vi "Handle Last Ack Core.vi"(4 "error in (no error)":errorcluster, 6 "Last Ack":refnum<class "Last Ack.lvclass">, 7 "Function in":refnum<class "Function.lvclass">) -> (0 "error out":errorcluster, 3 "Function out":refnum<class "Function.lvclass">)   [LabVIEW 2016, in "Function Actor.lvlib" / "Function.lvclass"]
doc: "(<B>Filename</B>: Actor Framework.lvlib:Actor.lvclass:Handle Last Ack Core.vi)\n\nDefines how the caller actor responds to the Last Ack message from a nested actor. The Last Ack message is the final message a nested actor sends to its caller before it shuts down. The message contains information about the final state of the nested actor.\n\nBy default, this method does nothing except return any error the nested actor sent. A descendant class may override this method to define behavior."
uses:
  <userlib>/Common Components/Function Actor/Function.lvclass
  <vilib>/ActorFramework/LastAck/Last Ack.lvclass
  <vilib>/ActorFramework/LastAck/Last Ack.lvclass/Last Ack.ctl
  <userlib>/Configuration Dialog Actor/Configuration.lvclass
  <userlib>/Configuration Dialog Actor/Configuration.lvclass/Configuration.ctl
  <userlib>/Common Components/Function Actor/Function.lvclass/Function.ctl
  <vilib>/ActorFramework/Actor/Actor.lvclass
  <userlib>/Common Components/Controller/Controller.lvclass
  C:/Program Files (x86)/National Instruments/LabVIEW 2016/vi.lib/ActorFramework/Actor/Actor.lvclass
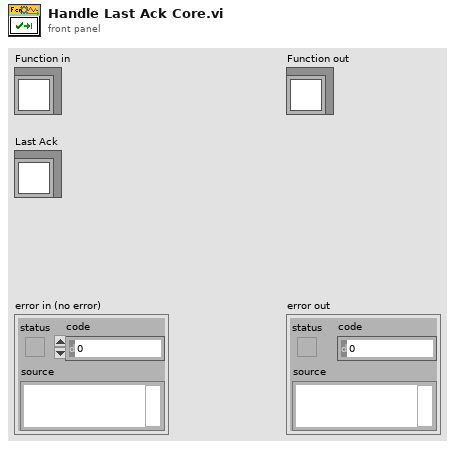
[diagram p1: front panel]
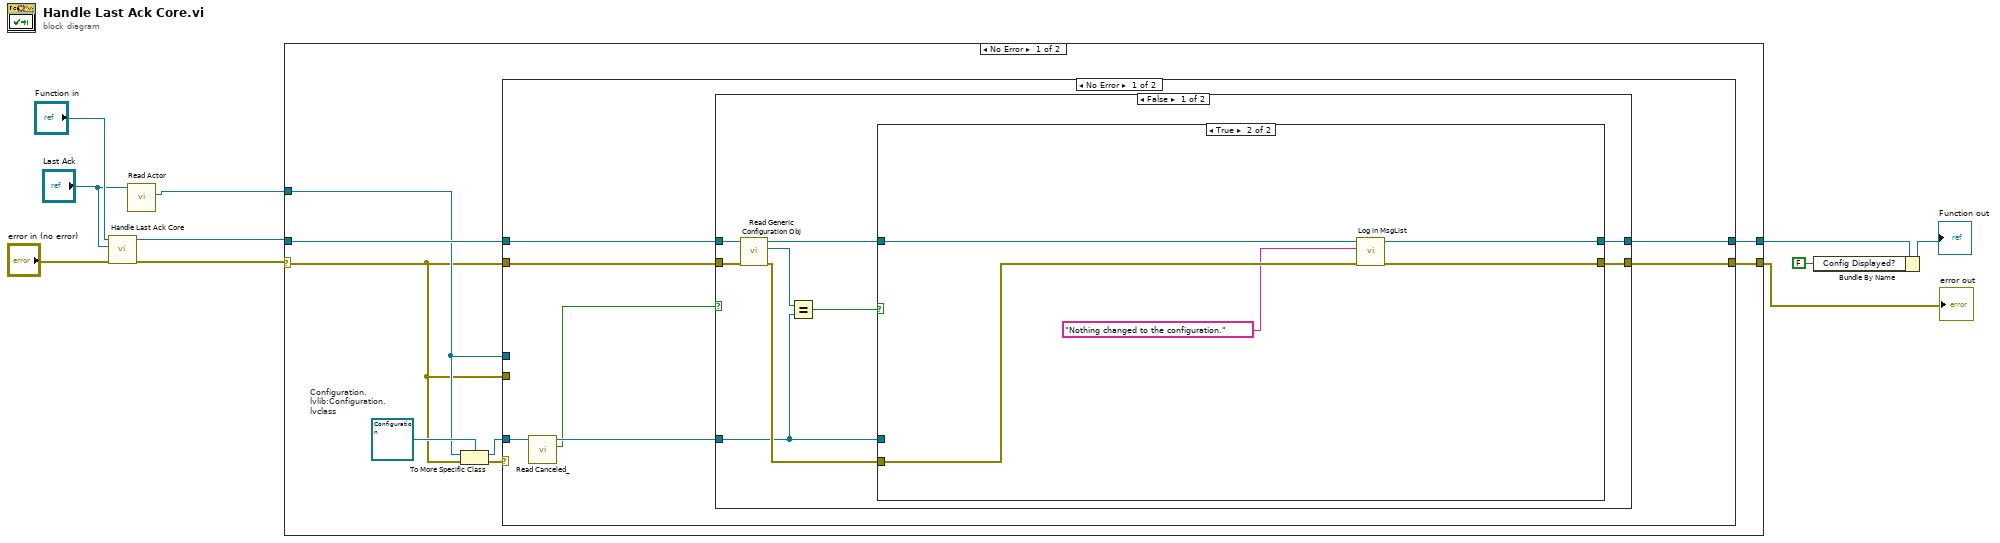
[diagram p0: block diagram]
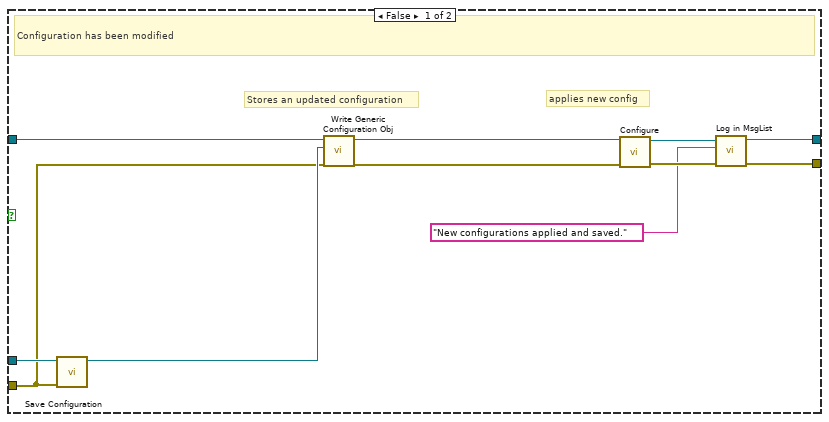
[diagram p2: hidden frame]
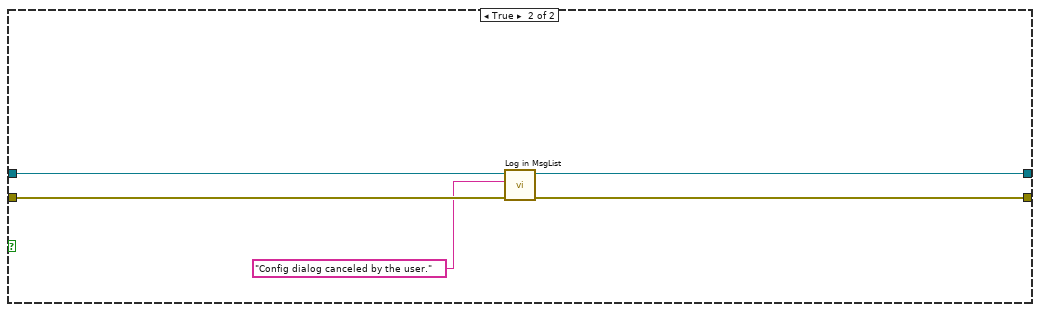
[diagram p3: hidden frame]
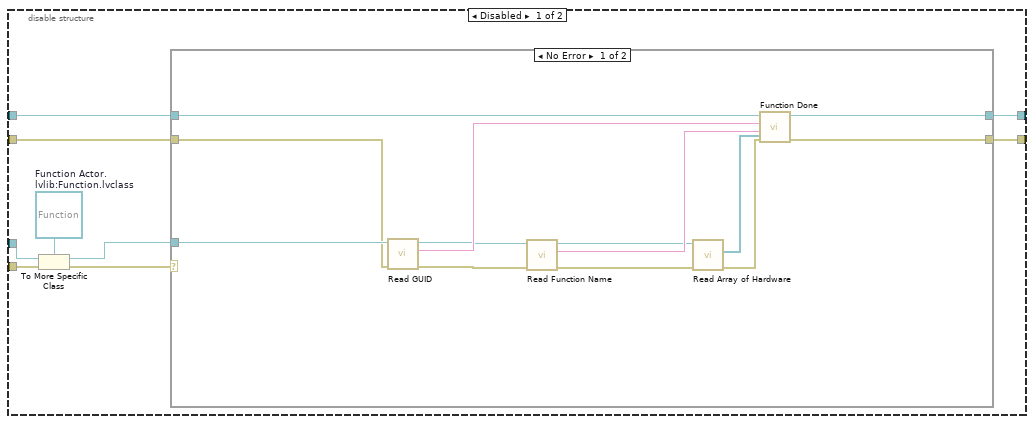
[diagram p5: hidden frame]
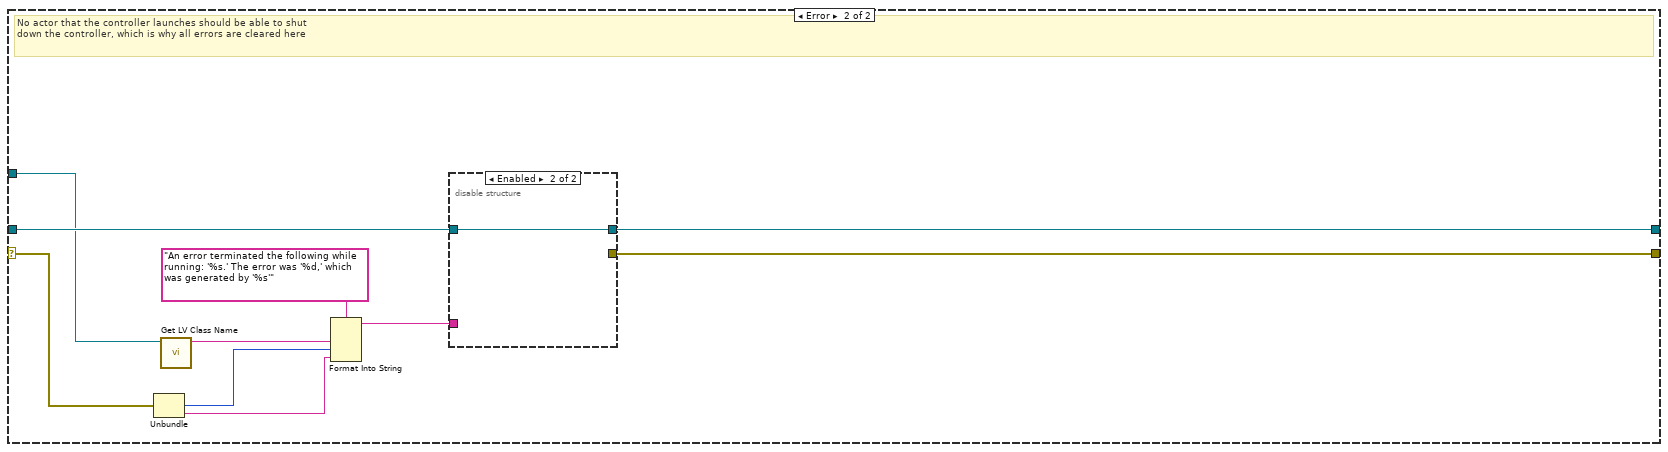
[diagram p7: hidden frame]
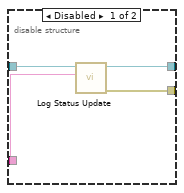
[diagram p8: hidden frame]
diagram:
  n1 = call-parent "Handle Last Ack Core.vi"("error in (no error)"="error in (no error)", "Last Ack"="Last Ack", "Actor in"="Function in") -> ("error out"=w5:errorcluster, "Actor out"=w6:refnum<class "Function.lvclass">)  [unwired: 3 in]
  n2 = call <vilib>:"Read Actor.vi"("Last Ack"="Last Ack") -> ("Actor"=w7:refnum<class "Actor.lvclass">)  [unwired: 10 in]
  n3 = case shown="No Error" w5 {
    selector: w5 -> [w11 w92]
    tunnel: [w18 w95] -> w3
    tunnel: [w17 w94] -> w4
    tunnel: w6 -> [w16 w96]
    tunnel: w7 -> [w12 w88]
    frame No Error {
      w13 = refnum<class "Configuration.lvclass"> refnum  # Configuration.lvlib:Configuration.lvclass
      n4 = To More Specific Class(target class=w13, reference=w12, error in=w11) -> (specific class reference=w15:refnum<class "Configuration.lvclass">, error out=w14:errorcluster)
      n5 = case shown="No Error" w14 {
        tunnel: [w21 w56] -> w18
        tunnel: [w25 w55] -> w17
        tunnel: w16 -> [w24 w58]
        tunnel: w15 -> [w22 _]
        tunnel: w11 -> [w23 w57]
        tunnel: w12 -> [_ w60]
        tunnel: w11 -> [_ w59]
        frame No Error {
          n6 = call <vilib>:"Read Canceled_.vi"("Configuration in"=w22) -> ("Canceled?"=w19:bool, "Configuration out"=w20:refnum<class "Configuration.lvclass">)  [unwired: 8 in, 1 out]
          n7 = case shown="False" w19 {
            tunnel: [w34 w53] -> w25
            tunnel: w24 -> [w33 w52]
            tunnel: w23 -> [w29 w54]
            tunnel: [w27 w51] -> w21
            tunnel: w20 -> [w26 _]
            frame False {
              n8 = call <userlib>:"Read Generic Configuration Obj.vi"("error in (no error)"=w29, "Function in"=w33) -> ("error out"=w32:errorcluster, "Configuration.lvlib:Configuration.lvclass"=w31:refnum<class "Configuration.lvclass">, "Function out"=w28:refnum<class "Function.lvclass">)  [unwired: 7 in]
              n9 = Equal?(x=w31, y=w26) -> (x = y?=w30:bool)
              n10 = case shown="True" w30 {
                tunnel: w26 -> [w44 _]
                tunnel: w32 -> [w40 w49]
                tunnel: w28 -> [w42 w47]
                tunnel: [w36 w46] -> w27
                tunnel: [w38 w48] -> w34
                frame False {
                  # "applies new config"
                  # "Stores an updated configuration"
                  # "Configuration has been modified"
                  n11 = call <userlib>:"Save Configuration.vi"("error in (no error)"=w40, "Configuration in"=w44) -> ("Configuration out"=w43:refnum<class "Configuration.lvclass">)  [unwired: 7 in, 2 out]
                  n12 = call <userlib>:"Write Generic Configuration Obj.vi"("Configuration.lvlib:Configuration.lvclass"=w43, "Function in"=w42) -> ("Function out"=w41:refnum<class "Function.lvclass">)  [unwired: 8 in, 1 out]
                  n13 = call-dynamic "Configure.vi"("error in (no error)"=w40, "Function in"=w41) -> ("error out"=w39:errorcluster, "Function out"=w37:refnum<class "Function.lvclass">)  [unwired: 8 in]
                  n14 = call-dynamic "Log in MsgList.vi"("error in (no error)"=w39, "Msg"="New configurations applied and saved.", "Function in"=w37) -> ("error out"=w38:errorcluster, "Function out"=w36:refnum<class "Function.lvclass">)  [unwired: 7 in]
                }
                frame True {
                  n15 = call-dynamic "Log in MsgList.vi"("error in (no error)"=w49, "Msg"="Nothing changed to the configuration.", "Function in"=w47) -> ("error out"=w48:errorcluster, "Function out"=w46:refnum<class "Function.lvclass">)  [unwired: 7 in]
                }
              }
            }
            frame True {
              n16 = call-dynamic "Log in MsgList.vi"("error in (no error)"=w54, "Msg"="Config dialog canceled by the user.", "Function in"=w52) -> ("error out"=w53:errorcluster, "Function out"=w51:refnum<class "Function.lvclass">)  [unwired: 7 in]
            }
          }
        }
        frame Error {
          n17 = disable-structure shown="Enabled" {
            disable-tunnel: w60 -> [w69 _]
            disable-tunnel: w59 -> [w68 _]
            disable-tunnel: w58 -> [w64 w86]
            disable-tunnel: w57 -> [w63 w85]
            disable-tunnel: [w62 w86] -> w56
            disable-tunnel: [w61 w85] -> w55
            frame Disabled {
              w67 = refnum<class "Function.lvclass"> refnum  # Function Actor.lvlib:Function.lvclass
              n18 = To More Specific Class(target class=w67, reference=w69, error in=w68) -> (specific class reference=w65:refnum<class "Function.lvclass">, error out=w66:errorcluster)
              n19 = case shown="No Error" w66 {
                tunnel: w65 -> [w76 _]
                tunnel: w64 -> [w82 w84]
                tunnel: w63 -> [w72 w83]
                tunnel: [w81 w84] -> w62
                tunnel: [w80 w83] -> w61
                frame No Error {
                  n20 = call <userlib>:"Read GUID.vi"("error in (no error)"=w72, "Function in"=w76) -> ("error out"=w71:errorcluster, "GUID"=w78:string, "Function out"=w75:refnum<class "Function.lvclass">)  [unwired: 7 in]
                  n21 = call <userlib>:"Read Function Name.vi"("error in (no error)"=w71, "Function in"=w75) -> ("error out"=w70:errorcluster, "Function Name"=w77:string, "Function out"=w74:refnum<class "Function.lvclass">)  [unwired: 7 in]
                  n22 = call <userlib>:"Read Array of Hardware.vi"("error in (no error)"=w70, "Function in"=w74) -> ("error out"=w73:errorcluster, "Array of Hardware"=w79:refnum<class "Hardware.lvclass">[])  [unwired: 7 in, 1 out]
                  n23 = call-dynamic "Function Done.vi"("Array of Hardware"=w79, "error in (no error)"=w73, "Function Name"=w77, "GUID"=w78, "Controller in"=w82) -> ("error out"=w80:errorcluster, "Controller out"=w81:refnum<class "Controller.lvclass">)  [unwired: 5 in]
                }
                frame Error {
                }
              }
            }
            frame Enabled {
            }
          }
        }
      }
    }
    frame Error {
      # "No actor that the controller launches should be able to shut\ndown the controller, which is why all errors are cleared here"
      n24 = Unbundle(w92) -> ("code"=w90:i32, "source"=w89:string)  [unwired: 1 out]
      n25 = call <vilib>:"Get LV Class Name.vi"("object"=w88) -> ("class name"=w87:string)  [unwired: 9 in, 1 out]
      n26 = Format Into String(format string="An error terminated the following while running: '%s.' The error was '%d,' which was generated by '%s'", w87, w90, w89) -> (resulting string=w93:string)  [unwired: 2 in, 1 out]
      n27 = disable-structure shown="Enabled" {
        disable-tunnel: w96 -> [w100 w101]
        disable-tunnel: [w99 w101] -> w95
        disable-tunnel: [w98 _] -> w94
        disable-tunnel: w93 -> [w97 _]
        frame Disabled {
          n28 = call-dynamic "Log Status Update.vi"("String"=w97, "Controller in"=w100) -> ("error out"=w98:errorcluster, "Controller out"=w99:refnum<class "Controller.lvclass">)  [unwired: 8 in]
        }
        frame Enabled {
        }
      }
    }
  }
  "error out" <- w4
  n29 = Bundle By Name(cluster=w3, "Config Displayed?"=FALSE) -> (→"Function out":refnum<class "Function.lvclass">)
